vi "GetPathFromName.vi"(0 "Experience ID":string="TestOK\nTest") -> (1 "Error out":errorcluster={"status"=TRUE, "code"=2, "source"="incorrect path for Experience ID"}, 2 "VI_Path":path)   [LabVIEW 2015]
uses:
  Configuration/Global_Configurations.vi
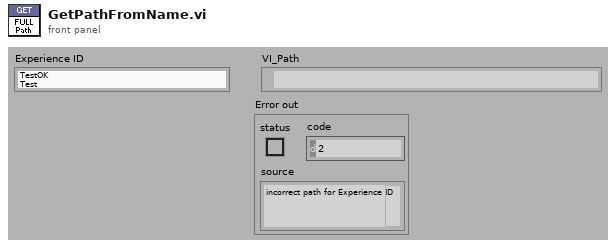
[diagram p1: front panel]
types:
  T1 = cluster{"Path":path, "Name":string, "Authors":string, "Keywords":string, "Description":string, "Cameras":cluster{"Base URL":string, "Path":string, "Name":string}[], "Delta":dbl, "Sampled Variable":string}[]
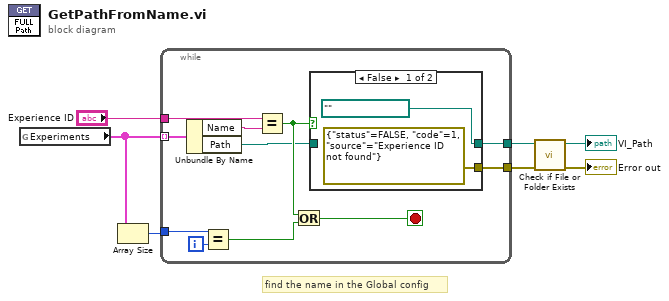
[diagram p0: block diagram]
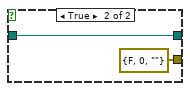
[diagram p2: hidden frame]
diagram:
  # "find the name in the Global config"
  n1 = global read "Global_Configurations.vi" "Experiments"() -> (w7:T1)
  n2 = Array Size(array=w7) -> (size(s)=w6:i32)
  n3 = while {
    tunnel: w7 -> [w18] mode=indexing
    tunnel: "Experience ID" -> [w17]
    tunnel: w6 -> [w15]
    tunnel: [w11] -> w4
    tunnel: [w9] -> w3
    i -> [w16]
    stop <- w13 stop-if-true
    n4 = Unbundle By Name(w18) -> ("Name"=w14:string, "Path"=w8:path)
    n5 = Equal?(x=w15, y=w16) -> (x = y?=w12:bool)
    n6 = Equal?(x=w17, y=w14) -> (x = y?=w10:bool)
    n7 = Or(x=w10, y=w12) -> (x .or. y?=w13:bool)
    n8 = case shown="False" w10 {
      tunnel: w8 -> [_ w22]
      tunnel: [path "" ("Path") w22] -> w11
      tunnel: [errorcluster {"status"=FALSE, "code"=1, "source"="Experience ID not found"} ("error in (no error)") errorcluster {"status"=FALSE, "code"=0, "source"=""} ("error in (no error)")] -> w9
      frame False {
      }
      frame True {
      }
    }
  }
  n9 = call <vilib>:"Check if File or Folder Exists.vi"("error in (no error)"=w3, "path"=w4) -> ("error out"=→"Error out":errorcluster, "dup path"=→"VI_Path":path)  [unwired: 8 out]
